vi "tutorial 3.vi"() -> ()   [LabVIEW 2022 SP3]
panel:
  in  "stop":bool
  out "return value":dbl
  in  "input2":dbl
  in  "input1":dbl
  in  "multiple functions":string(combo)
  in  "Python version":string
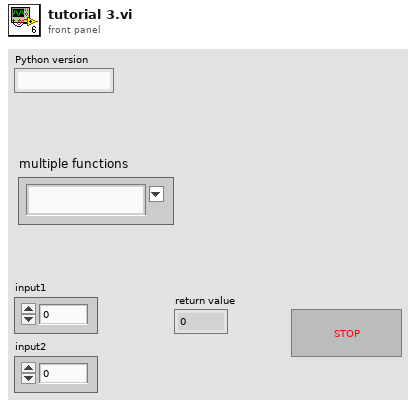
[diagram p1: front panel]
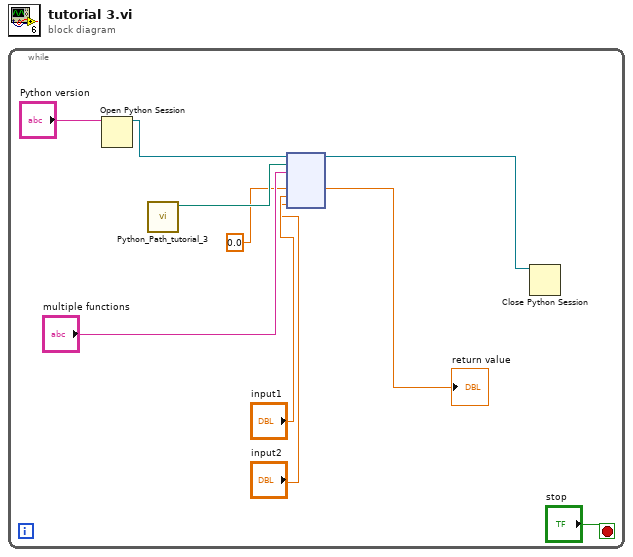
[diagram p0: block diagram]
diagram:
  n1 = while {
    stop <- "stop" stop-if-true
    n2 = Open Python Session(python version="Python version") -> (session out=w9:refnum<k35>)  [unwired: 2 in, 1 out]
    n3 = call "Python_Path_tutorial_3.vi"() -> ("appended path"=w7:path)  [unwired: 11 in]
    n4 = node(w9, w7, "multiple functions", 0.0, "input1", "input2") -> (w8:refnum<k35>, →"return value":dbl)  [unwired: 3 in, 3 out]
    n5 = Close Python Session(session in=w8) -> ()  [unwired: 1 in, 1 out]
  }
